vi "test Import Version 1.1 Bus Controller Address.vi"(8 "error in":errorcluster, 11 "TestCase in":refnum<class "1553 Parameters Import.lvclass">) -> (0 "error out":errorcluster, 3 "TestCase out":refnum<class "1553 Parameters Import.lvclass">)   [LabVIEW 2020, in "1553 Parameters Import.lvclass"]
uses:
  1553 Parameters Import.lvclass
  <vilib>/addons/_JKI Toolkits/VI Tester/TestCase.llb/TestCase.lvclass
  Import/MIL-STD 1553 Import.lvlib
  C:/Program Files (x86)/National Instruments/LabVIEW 2020/vi.lib/addons/_JKI Toolkits/VI Tester/TestCase.llb/TestCase.lvclass
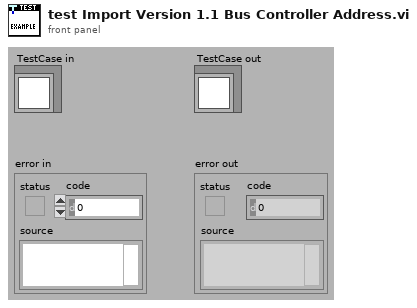
[diagram p1: front panel]
types:
  T1 = typedef "1553 Channel.ctl" = cluster{"HW channel":u16, "bus controller address":i16, "terminal addresses":T2[], "terminal names":string[], "acyclic frame names":string[], "messages":T3[]}
  T2 = typedef "Address.ctl" = u16
  T3 = typedef "Message Definition.ctl" = cluster{"name":string, "message type":T4, "endpoint Tx":T5, "endpoint Rx":T5, "create timestamp channel":bool, "mode code":u16, "number of words":u16, "parameters":cluster{"name":string, "default value":dbl, "unit":string, "parameter definition":T6}[]}
  T4 = typedef "Message Type.ctl" = string
  T5 = typedef "Terminal Endpoint.ctl" = cluster{"terminal address":T2, "subaddress":T2}
  T6 = typedef "Parameter Definition.ctl" = cluster{"start index":i32, "size (bits)":i32, "encoding":enum16{"BNR", "BCD", "Discrete"}, "signed":bool, "multiplier":dbl, "offset":dbl}
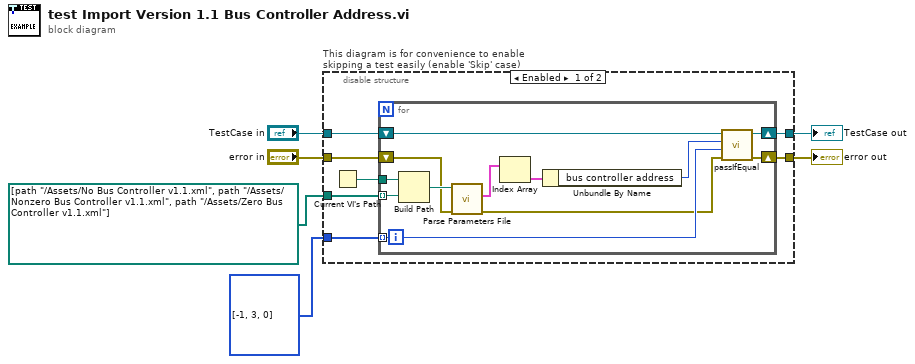
[diagram p0: block diagram]
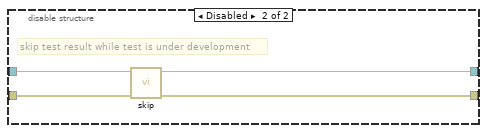
[diagram p2: hidden frame]
diagram:
  n1 = disable-structure "This diagram is for convenience to enable skipping a test easily (enable 'Skip' case)" shown="Enabled" {
    disable-tunnel: "TestCase in" -> [w13 w29]
    disable-tunnel: [w12 w27] -> w3
    disable-tunnel: [w9 w28] -> w5
    disable-tunnel: "error in" -> [w11 w26]
    disable-tunnel: i16[] [-1, 3, 0] ("bus controller") -> [w8 _]
    disable-tunnel: path[] [path "../Assets/No Bus Controller v1.1.xml", path "../Assets/Nonzero Bus Controller v1.1.xml", path "../Assets/Zero Bus Controller v1.1.xml"] -> [w7 _]
    frame Enabled {
      n2 = Current VI's Path() -> (path=w10:path)
      n3 = for {
        shift-right: [w22] -> w12
        shift-left: w13 -> [w23]
        shift-right: [w21] -> w9
        shift-left: w11 -> [w20]
        tunnel: w10 -> [w24]
        tunnel: w8 -> [w17] mode=indexing
        tunnel: w7 -> [w14] mode=indexing
        n4 = Build Path(base path=w24, name or relative path=w14) -> (appended path=w25:path)
        n5 = call "Parse Parameters File.vi"("error in"=w20, "path to XML document"=w25) -> ("error out"=w15:errorcluster, "1553 channels"=w19:T1[])  [unwired: 7 in, 1 out]
        n6 = Index Array(array=w19) -> (element=w18:T1)  [unwired: 1 in]
        n7 = Unbundle By Name(w18) -> ("bus controller address"=w16:i16)
        n8 = call-dynamic "passIfEqual.vi"("error in (no error)"=w15, "y"=w17, "x"=w16, "TestCase in"=w23) -> ("error out"=w21:errorcluster, "TestCase out"=w22:refnum<class "1553 Parameters Import.lvclass">)  [unwired: 6 in]
      }
    }
    frame Disabled {
      # "skip test result while test is under development"
      n9 = call <vilib>:"skip.vi"("error in (no error)"=w26, "TestCase in"=w29) -> ("error out"=w28:errorcluster, "TestCase out"=w27:refnum<class "1553 Parameters Import.lvclass">)  [unwired: 8 in]
    }
  }
  "error out" <- w5
  "TestCase out" <- w3
